vi "Write_output_file.vi"(0 "Output filename":path, 1 "Header":string, 2 "Template Filename":path, 5 "Channel Names":string[](array[string]), 7 "Data":string[][](array[string]), 9 "Desired Columns":i32[](array[numeric])=[0, 1, 2, 3, 4, 5, 6, 7, 8, 9, 10, 11, 12, 13, 14, 15, 16, 17, 18, 19, 20, 21, 22, 23, 24, 25, 26, 27, 28, 29, 30, 31, 32, 33, 34, 35, 36, 37, 38, 39, 40, 41, 42, 43, 44, 45, 46, 47, 48, 49, 50, 51, 52, 53, 54, 55, 56, 57, 58, 59, 60, 61, 62, 63, 64, 65, 66, 67, 68, 69, 70, 71, 72, 73, 74, 75, 76, 77, 78, 79, 80, 81, 82, 83, 84, 85, 86, 87, 88, 89, 90, 91, 92, 93, 94, 95, 96, 97, 98, 99, 100, 101, 102, 103, 104, 105, 106, 107, 108, 109, 110, 111, 112, 113, 114, 115, 116, 117, 118, 119, 120, 121, 122, 123, 124, 125, 126, 127, 128, 129, 130, 131, 132, 133, 134, 135, 136, 137, 138, 139, 140, 141, 142, 143, 144, 145, 146, 147, 148, 149, 150, 151, 152, 153, 154, 155, 156, 157, 158, 159, 160, 161, 162, 163, 164, 165, 166, 167, 168, 169, 170, 171, 172, 173, 174, 175, 176, 177, 178, 179, 180, 181, 182, 183, 184, 185, 186, 187, 188, 189, 190, 191, 192, 193, 194, 195, 196, 197, 198, 199, 200, 201, 202, 203, 204, 205, 206, 207, 208, 209, 210, 211, 212, 213, 214, 215, 216, 217, 218, 219, 220, 221, 222, 223, 224, 225, 226, 227, 228, 229, 230, 231, 232, 233, 234], 11 "Simple Save?":bool, 12 "Save Plotted rows only?":bool, 13 "Summarise mode":T2(ring), 14 "Grouping info":T3[](array[typedef]), 15 "Channels to Tabulate in header":i32[](listbox)) -> (4 "Output filename Out":path)   [LabVIEW 2015]
uses:
  Controls/Group_Binning.ctl
  Results_plotter_Global.vi
panel:
  out "Which Button?":T1(ring)=enum."Center Button"
  out "Table Values":string[][](array[string])
  out "Table Names":string[](array[string])
  out "Table":string
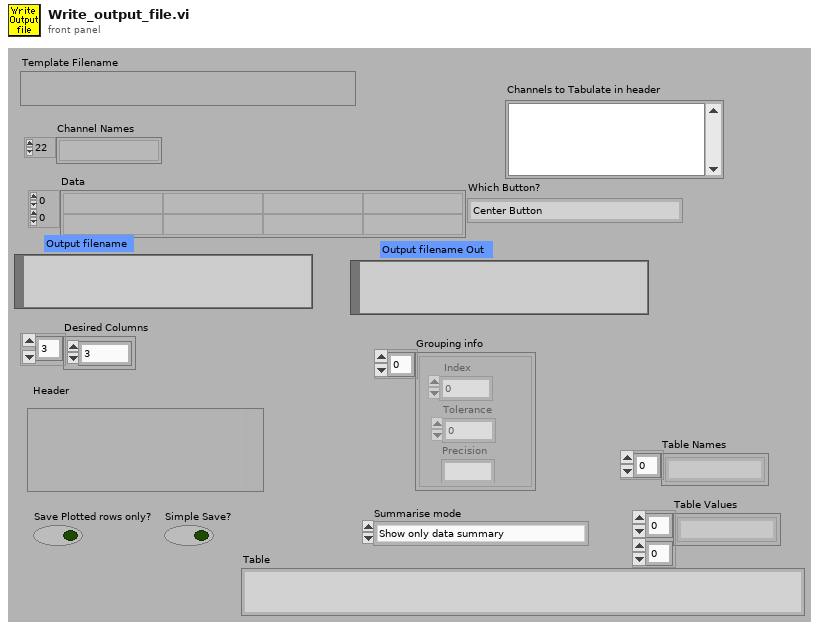
[diagram p1: front panel]
types:
  T1 = enum16{"Left Button", "Center Button", "Right Button", "Window Close"}
  T2 = enum16{"Show only data summary", "Show data summary", "No data summary"}
  T3 = typedef "Group_Binning.ctl" = cluster{"Index":i32, "Tolerance":dbl, "Precision":string}
  T4 = enum32{"existing file", "new file", "new or existing file", "existing dir", "new dir", "new or existing dir", "existing file (use LLBs)", "new file (use LLBs)", "new or existing file (use LLBs)", "new or existing file or directory (use LLBs)"}
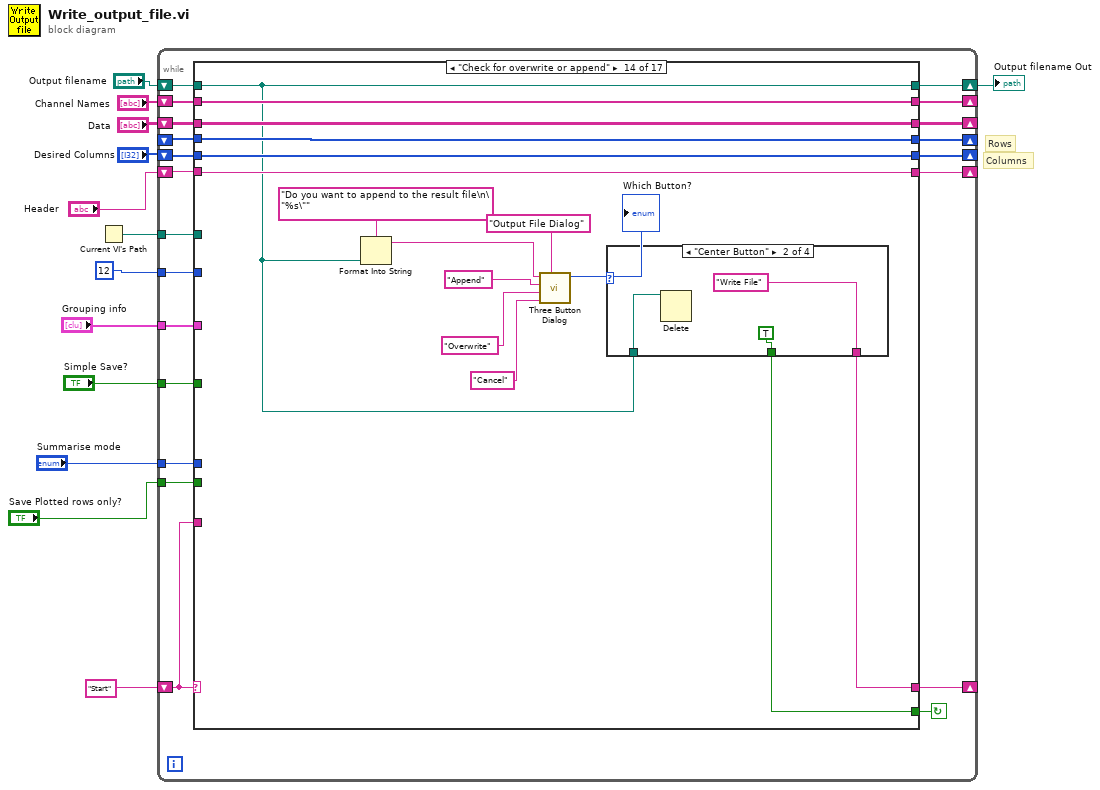
[diagram p0: block diagram]
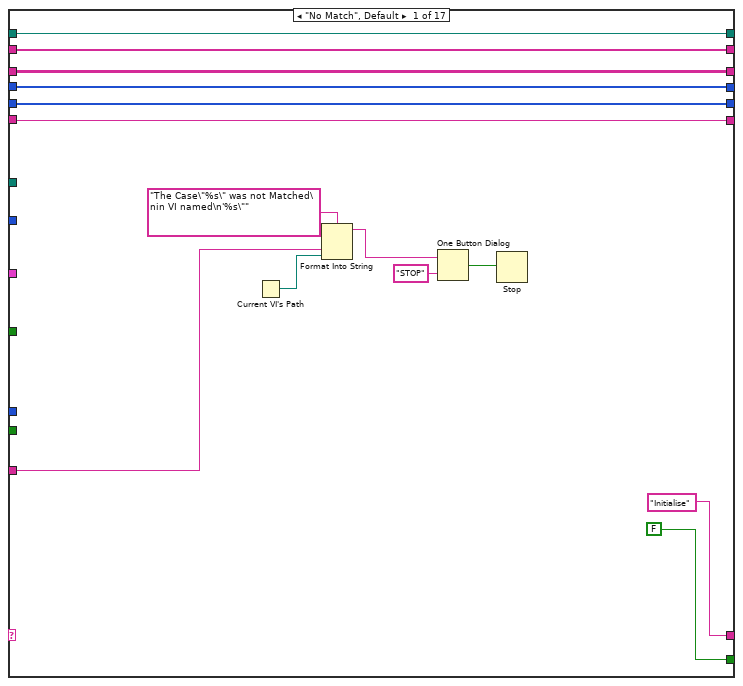
[diagram p2: hidden frame]
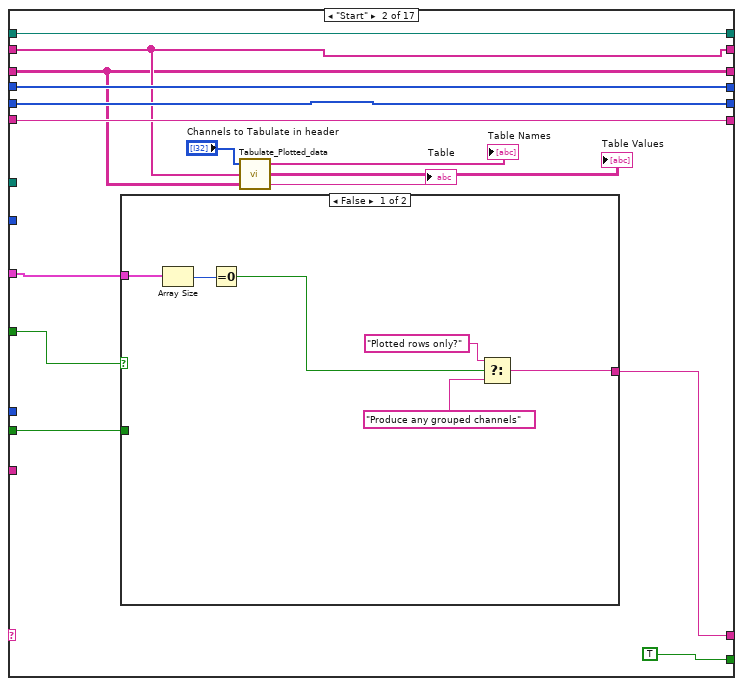
[diagram p3: hidden frame]
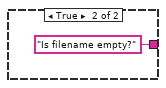
[diagram p4: hidden frame]
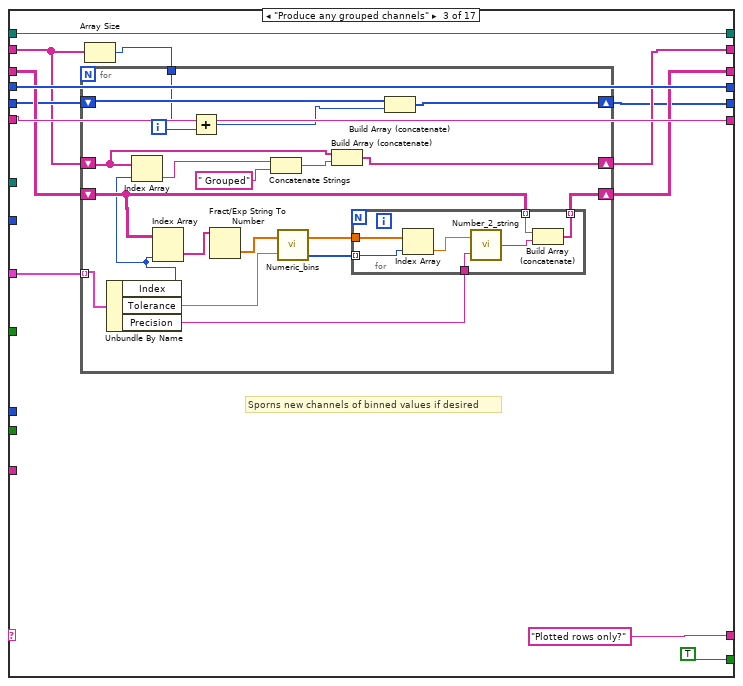
[diagram p5: hidden frame]
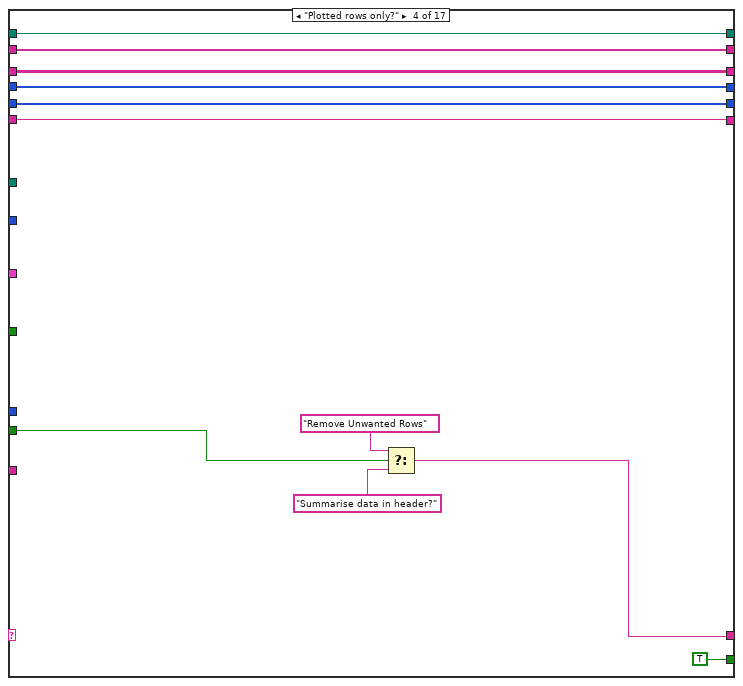
[diagram p6: hidden frame]
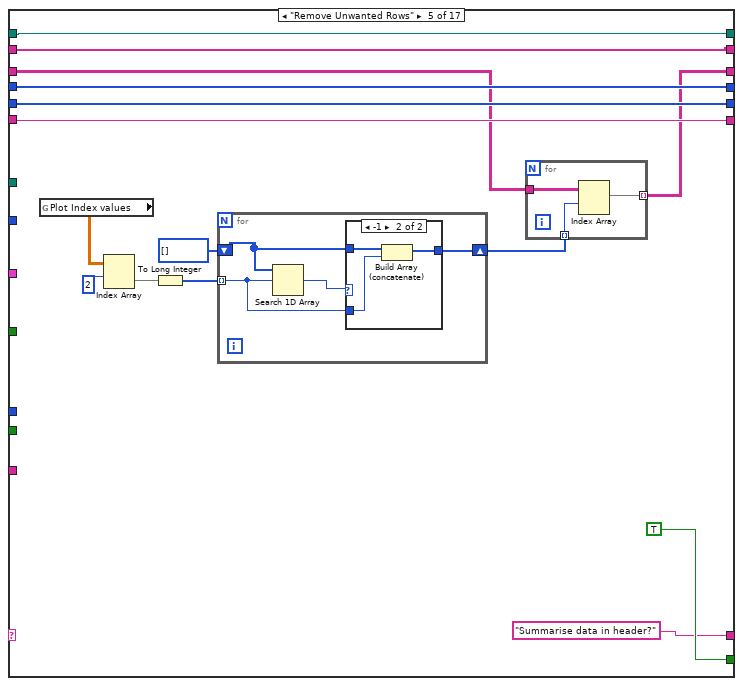
[diagram p7: hidden frame]
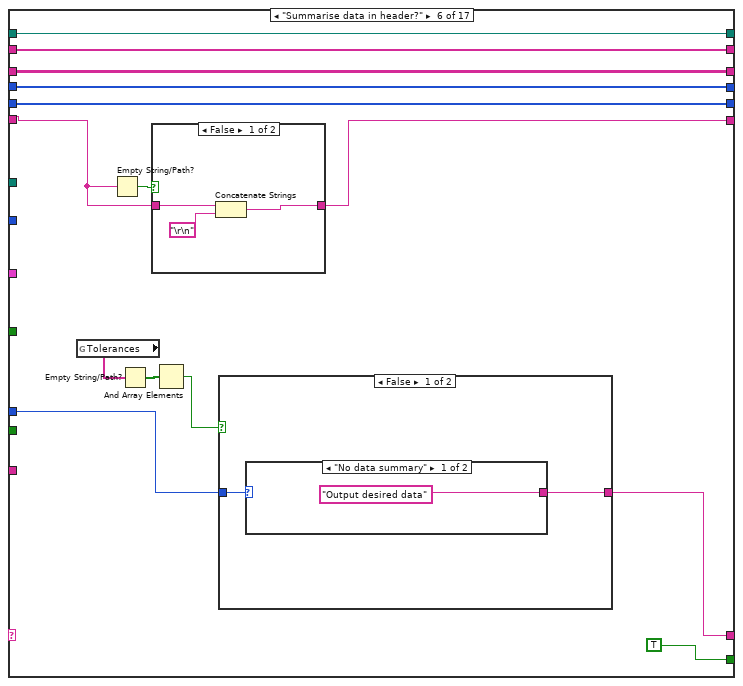
[diagram p9: hidden frame]
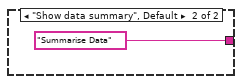
[diagram p10: hidden frame]
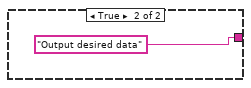
[diagram p11: hidden frame]
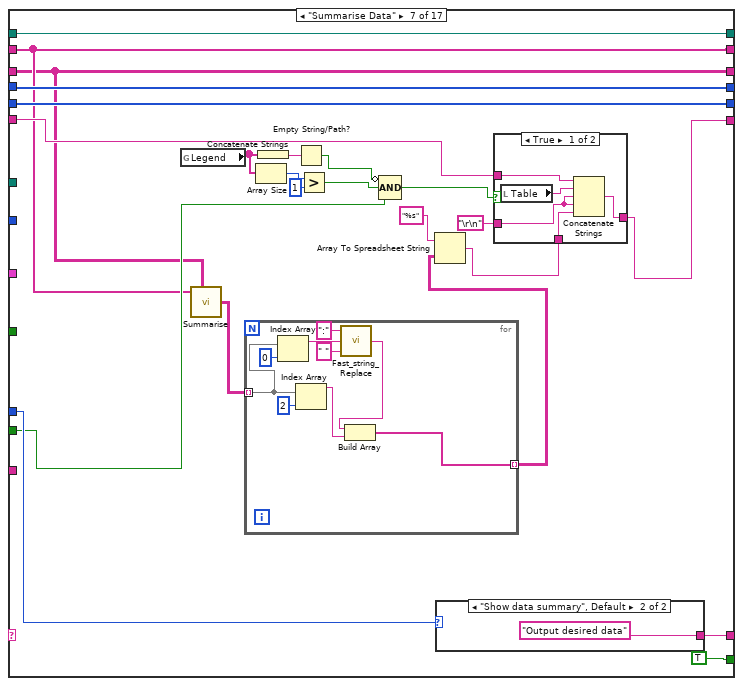
[diagram p13: hidden frame]
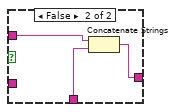
[diagram p14: hidden frame]
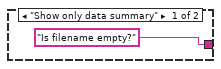
[diagram p15: hidden frame]
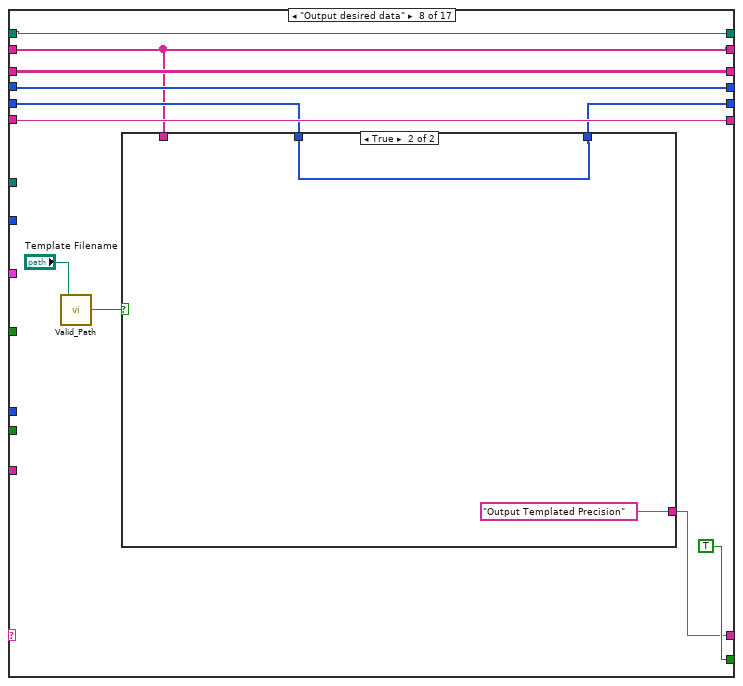
[diagram p16: hidden frame]
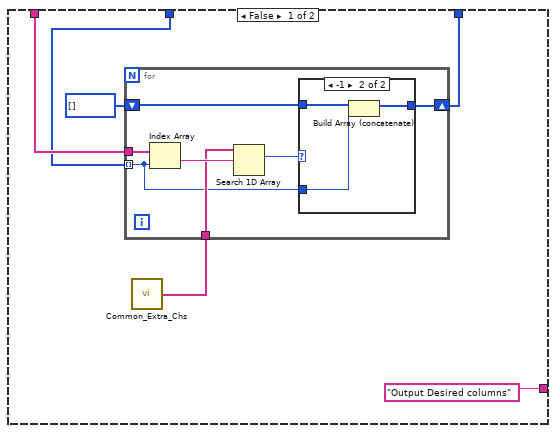
[diagram p17: hidden frame]
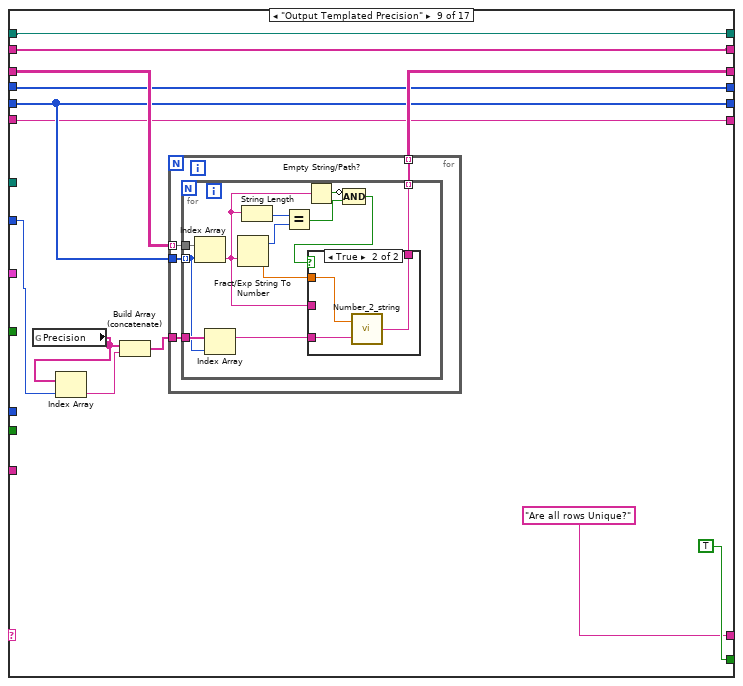
[diagram p19: hidden frame]
diagram:
  # "Columns"
  # "Rows"
  n1 = Current VI's Path() -> (path=w11:path)
  n2 = while {
    shift-left: "Header" -> [w24]
    shift-right: [w27] -> _
    shift-left: "Desired Columns" -> [w26]
    shift-right: [w25] -> _
    shift-left: _ -> [w28]
    shift-right: [w29] -> _
    shift-left: "Data" -> [w31]
    shift-right: [w30] -> _
    shift-left: "Start" -> [w32]
    shift-right: [w33] -> _
    tunnel: w11 -> [w23]
    shift-right: [w22] -> w10
    shift-left: "Output filename" -> [w21]
    shift-right: [w19] -> _
    shift-left: "Channel Names" -> [w20]
    tunnel: "Simple Save?" -> [w18]
    tunnel: 12 ("disabled index (col)") -> [w17]
    tunnel: "Grouping info" -> [w16]
    tunnel: "Summarise mode" -> [w15]
    tunnel: "Save Plotted rows only?" -> [w14]
    stop <- w34 continue-if-true
    n3 = case shown="\"Check for overwrite or append\"" w32 {
      tunnel: [FALSE TRUE TRUE TRUE ("cancelled") TRUE TRUE TRUE TRUE TRUE TRUE TRUE TRUE w349 w366 TRUE ("cancelled") FALSE ("cancelled") FALSE] -> w34
      tunnel: ["Initialise" w60 "Plotted rows only?" w112 "Summarise data in header?" w159 w189 w220 "Are all rows Unique?" "Is filename empty?" w296 "Is filename empty?" w350 w367 "Write File" "End" "End"] -> w33
      tunnel: w32 -> [w43 _ _ _ _ _ _ _ _ _ _ _ _ _ _ _ _]
      tunnel: w31 -> [w40 w53 w79 w116 w128 w155 w172 w217 w254 w283 w303 w339 w354 w376 w396 w410 w436]
      tunnel: [w40 w53 w77 w116 w127 w155 w172 w217 w253 w278 w303 w338 w354 w376 w396 w410 w436] -> w30
      tunnel: [w39 w62 w82 w115 w135 w160 w192 w222 w252 w282 w302 w337 w355 w377 w399 w419 w443] -> w29
      tunnel: w28 -> [w39 w62 w82 w115 w135 w160 w192 w222 w252 w282 _ w337 w355 w377 w399 w419 w443]
      tunnel: [w37 w61 w80 w113 w134 w151 w190 w221 w250 w280 w294 w334 w356 w378 w391 w420 w435] -> w27
      tunnel: w26 -> [w38 w57 w75 w114 w133 w154 w191 w219 w251 w281 w295 w335 w357 w379 w394 w401 w442]
      tunnel: [w38 w57 w72 w114 w133 w154 w191 w218 w251 w281 w295 w335 w357 w379 w394 w401 w442] -> w25
      tunnel: w24 -> [w37 w61 w80 w113 w134 w152 w174 w221 w250 w280 w294 w334 w356 w378 w389 w420 w435]
      tunnel: w23 -> [_ _ _ _ _ _ _ _ _ _ _ _ _ _ _ _ _]
      tunnel: [w36 w59 w81 w118 w123 w158 w188 w216 w248 w277 w293 w333 w353 w365 w393 w406 w438] -> w22
      tunnel: w21 -> [w36 w59 w81 w118 w123 w158 w188 w216 w248 w277 w293 w333 w346 w365 w393 w406 w438]
      tunnel: w20 -> [w35 w54 w74 w117 w122 w156 w173 w215 w247 w276 w292 w332 w348 w374 w395 w403 w439]
      tunnel: [w35 w54 w76 w117 w122 w156 w173 w215 w247 w276 w292 w332 w348 w374 w395 w403 w439] -> w19
      tunnel: w18 -> [_ w58 _ _ _ _ _ _ _ _ _ _ _ _ _ w402 w437]
      tunnel: w17 -> [_ _ _ _ _ _ _ _ w246 _ _ _ _ _ _ _ _]
      tunnel: w16 -> [_ w51 w78 _ _ _ _ _ _ _ _ _ _ _ _ _ _]
      tunnel: w15 -> [_ _ _ _ _ w157 w187 _ _ _ _ _ _ _ _ _ w434]
      tunnel: w14 -> [_ w56 _ w120 _ _ w186 _ _ _ _ _ _ _ _ _ _]
      frame "No Match", Default {
        n4 = Current VI's Path() -> (path=w42:path)
        n5 = Format Into String(format string="The Case\"%s\" was not Matched\nin VI named\n'%s\"" ("Format String"), w43, w42) -> (resulting string=w46:string)  [unwired: 2 in, 1 out]
        n6 = One Button Dialog(message=w46, button name ("OK")="STOP") -> (true=w44:bool)
        n7 = Stop(stop? (T)=w44) -> ()
      }
      frame "Start" {
        n8 = case shown="False" w58 {
          tunnel: [w64 "Is filename empty?" ("f")] -> w60
          tunnel: w56 -> [_ _]
          tunnel: w51 -> [w68 _]
          frame False {
            n9 = Array Size(array=w68) -> (size(s)=w69:i32)
            n10 = Equal To 0?(x=w69) -> (x = 0?=w67:bool)
            n11 = Select(t="Plotted rows only?", s=w67, f="Produce any grouped channels") -> (s? t:f=w64:string)
          }
          frame True {
          }
        }
        n12 = call "Tabulate_Plotted_data.vi"("Data"=w53, "Channel Names"=w54, "Channels to Tabulate"="Channels to Tabulate in header") -> ("spreadsheet string"=→"Table":string, "Channel Values"=→"Table Values":string[][], "Channel Names"=→"Table Names":string[])
      }
      frame "Produce any grouped channels" {
        # "Sporns new channels of binned values if desired"
        n13 = Array Size(array=w74) -> (size(s)=w73:i32)
        n14 = for {
          shift-right: [w95] -> w77
          shift-left: w79 -> [w96]
          tunnel: w78 -> [w100] mode=indexing
          shift-right: [w89] -> w76
          shift-left: w74 -> [w90]
          shift-right: [w87] -> w72
          shift-left: w75 -> [w88]
          tunnel: w73 -> [w85]
          i -> [w86]
          n15 = Unbundle By Name(w100) -> ("Index"=w94:i32, "Tolerance"=w98:dbl, "Precision"=w97:string)
          n16 = Index Array(array=w90, index=w94) -> (element=w92:string)
          n17 = Index Array(array=w96, index (col)=w94) -> (element=w99:string[])  [unwired: 1 in]
          n18 = Add(x=w85, y=w86) -> (x+y=w84:i32)
          n19 = Fract/Exp String To Number(string=w99) -> (number=w103:dbl[])  [unwired: 4 out]
          n20 = Concatenate Strings(w92, " Grouped" ("string")) -> (w91:string)
          n21 = call "Numeric_bins.vi"("Values"=w103, "Tolerance"=w98) -> ("Bin Centres"=w102:dbl[], "Bin Index"=w101:i32[])  [unwired: 1 out]
          n22 = Build Array (concatenate)(w90, w91) -> (w89:string[])
          n23 = for {
            tunnel: w102 -> [w110]
            tunnel: w101 -> [w109] mode=indexing
            tunnel: [w106] -> w95 mode=indexing
            tunnel: w97 -> [w105]
            tunnel: w96 -> [w104] mode=indexing
            n24 = Index Array(array=w110, index=w109) -> (element=w108:dbl)
            n25 = call "Number_2_string.vi"("precision"=w105, "number"=w108) -> ("String"=w107:string)
            n26 = Build Array (concatenate)(w104, w107) -> (w106:string[])
          }
          n27 = Build Array (concatenate)(w88, w84) -> (w87:i32[])
        }
      }
      frame "Plotted rows only?" {
        n28 = Select(t="Remove Unwanted Rows" ("f"), s=w120, f="Summarise data in header?") -> (s? t:f=w112:string)
      }
      frame "Remove Unwanted Rows" {
        n29 = global read "Results_plotter_Global.vi" "Plot Index values"() -> (w132:dbl[][])
        n30 = Index Array(array=w132, index (row)=2 ("disabled index (col)")) -> (element=w131:dbl[])  [unwired: 1 in]
        n31 = To Long Integer(number=w131) -> (32bit integer=w130:i32[])
        n32 = for {
          shift-right: [w141] -> w126
          shift-left: i32[] [] -> [w142]
          tunnel: w130 -> [w140] mode=indexing
          n33 = Search 1D Array(1D array=w142, element=w140) -> (index of element=w143:i32)  [unwired: 1 out]
          n34 = case shown="-1" w143 {
            tunnel: w142 -> [w144 w147]
            tunnel: [w144 w146] -> w141
            tunnel: w140 -> [_ w145]
            frame 0, Default {
            }
            frame -1 {
              n35 = Build Array (concatenate)(w147, w145) -> (w146:i32[])
            }
          }
        }
        n36 = for {
          tunnel: w126 -> [w139] mode=indexing
          tunnel: w128 -> [w138]
          tunnel: [w137] -> w127 mode=indexing
          n37 = Index Array(array=w138, index (row)=w139) -> (element=w137:string[])  [unwired: 1 in]
        }
      }
      frame "Summarise data in header?" {
        n38 = global read "Results_plotter_Global.vi" "Tolerances"() -> (w150:string[])
        n39 = Empty String/Path?(string/path=w152) -> (empty?=w153:bool)
        n40 = Empty String/Path?(string/path=w150) -> (empty?=w149:bool[])
        n41 = case shown="False" w153 {
          tunnel: [w167 w170] -> w151
          tunnel: w152 -> [w168 w170]
          frame False {
            n42 = Concatenate Strings(w168, "\r\n") -> (w167:string)
          }
          frame True {
          }
        }
        n43 = And Array Elements(Boolean array=w149) -> (logical AND=w148:bool)
        n44 = case shown="False" w148 {
          tunnel: [w163 "Output desired data" ("t")] -> w159
          tunnel: w157 -> [w162 _]
          frame False {
            n45 = case shown="\"No data summary\"" w162 {
              tunnel: ["Output desired data" ("t") "Summarise Data"] -> w163
              frame "No data summary" {
              }
              frame "Show data summary", Default {
              }
            }
          }
          frame True {
          }
        }
      }
      frame "Summarise Data" {
        n46 = global read "Results_plotter_Global.vi" "Legend"() -> (w179:string[])
        n47 = call "Summarise.vi"("Channel Names"=w173, "Data"=w172) -> ("Summary"=w184:string[][])  [unwired: 2 in, 1 out]
        n48 = for {
          tunnel: w184 -> [w208] mode=indexing
          tunnel: [w202] -> w171 mode=indexing
          n49 = Index Array(array=w208, index=0) -> (element=w206:string)
          n50 = Index Array(array=w208, index=2) -> (element=w207:string)
          n51 = call "Fast_string_Replace.vi"("Replace match with:"=" ", "Input String"=w206, "regular expression"=":") -> ("Output String"=w203:string)  [unwired: 2 out]
          n52 = Build Array(w203, w207) -> (w202:string[])
        }
        n53 = Array Size(array=w179) -> (size(s)=w178:i32)
        n54 = Concatenate Strings(w179) -> (w181:string)
        n55 = Empty String/Path?(string/path=w181) -> (empty?=w176:bool)
        n56 = Greater?(x=w178, y=1) -> (0:w175:bool)
        n57 = Compound Arithmetic op=AND(invert w176, w175, w186) -> (w180:bool)
        n58 = Array To Spreadsheet String(array=w171, 3:"%s" ("format string")) -> (spreadsheet string=w183:string)  [unwired: 1 out]
        n59 = case shown="\"Show data summary\", Default" w187 {
          tunnel: ["Is filename empty?" "Output desired data"] -> w189
          frame "Show only data summary" {
          }
          frame "Show data summary", Default {
          }
        }
        n60 = case shown="True" w180 {
          tunnel: [w195 w200] -> w190
          tunnel: w174 -> [w198 w199]
          tunnel: w183 -> [w196 w201]
          tunnel: "\r\n" -> [w197 _]
          frame True {
            n61 = local read "Table"() -> (w194:string)
            n62 = Concatenate Strings(w198, w194, w197, w197, w196) -> (w195:string)
          }
          frame False {
            n63 = Concatenate Strings(w199, w201) -> (w200:string)
          }
        }
      }
      frame "Output desired data" {
        n64 = call "Valid_Path.vi"("Filename"="Template Filename") -> ("Valid Path?"=w213:bool)
        n65 = case shown="True" w213 {
          tunnel: ["Output Desired columns" "Output Templated Precision" ("f")] -> w220
          tunnel: w219 -> [w227 w241]
          tunnel: [w225 w241] -> w218
          tunnel: w215 -> [w228 _]
          frame False {
            n66 = call "Common_Extra_Chs.vi"() -> ("Common Extra Channels"=w224:string[])
            n67 = for {
              shift-right: [w230] -> w225
              shift-left: i32[] [] -> [w232]
              tunnel: w228 -> [w236]
              tunnel: w227 -> [w231] mode=indexing
              tunnel: w224 -> [w234]
              n68 = Index Array(array=w236, index=w231) -> (element=w235:string)
              n69 = Search 1D Array(1D array=w234, element=w235) -> (index of element=w233:i32)  [unwired: 1 out]
              n70 = case shown="-1" w233 {
                tunnel: w232 -> [w237 w240]
                tunnel: w231 -> [_ w239]
                tunnel: [w237 w238] -> w230
                frame 0, Default {
                }
                frame -1 {
                  n71 = Build Array (concatenate)(w240, w239) -> (w238:i32[])
                }
              }
            }
          }
          frame True {
          }
        }
      }
      frame "Output Templated Precision" {
        n72 = global read "Results_plotter_Global.vi" "Precision"() -> (w245:string[])
        n73 = Index Array(array=w245, index=w246) -> (element=w243:string)
        n74 = Build Array (concatenate)(w245, w243) -> (w244:string[])
        n75 = for {
          tunnel: w251 -> [w259]
          tunnel: w254 -> [w258] mode=indexing
          tunnel: w244 -> [w257]
          tunnel: [w256] -> w253 mode=indexing
          n76 = for {
            tunnel: w259 -> [w269] mode=indexing
            tunnel: w258 -> [w271]
            tunnel: w257 -> [w270]
            tunnel: [w263] -> w256 mode=indexing
            n77 = Index Array(array=w271, index=w269) -> (element=w262:string)
            n78 = Index Array(array=w270, index=w269) -> (element=w261:string)
            n79 = Fract/Exp String To Number(string=w262) -> (offset past number=w267:i32, number=w264:dbl)  [unwired: 3 out]
            n80 = String Length(string=w262) -> (length=w268:i32)
            n81 = Equal?(x=w268, y=w267) -> (x = y?=w265:bool)
            n82 = Empty String/Path?(string/path=w262) -> (empty?=w266:bool)
            n83 = Compound Arithmetic op=AND(invert w266, w265) -> (w260:bool)
            n84 = case shown="True" w260 {
              tunnel: w261 -> [_ w274]
              tunnel: w264 -> [_ w275]
              tunnel: [w272 w273] -> w263
              tunnel: w262 -> [w272 _]
              frame False {
              }
              frame True {
                n85 = call "Number_2_string.vi"("precision"=w274, "number"=w275) -> ("String"=w273:string)
              }
            }
          }
        }
      }
      frame "Output Desired columns" {
        n86 = for {
          tunnel: w281 -> [w287]
          tunnel: w283 -> [w286] mode=indexing
          tunnel: [w285] -> w278 mode=indexing
          n87 = for {
            tunnel: w287 -> [w289] mode=indexing
            tunnel: w286 -> [w290]
            tunnel: [w288] -> w285 mode=indexing
            n88 = Index Array(array=w290, index=w289) -> (element=w288:string)
          }
        }
      }
      frame "Are all rows Unique?" {
        n89 = for {
          shift-right: [w309] -> _
          shift-left: _ -> [w308]
          tunnel: w303 -> [w311] mode=indexing
          shift-right: [w307] -> w302
          shift-left: _ -> [w306]
          tunnel: [w305] -> w299
          i -> [w305]
          n90 = Array To Spreadsheet String(array=w311, 3:"%s" ("format string")) -> (spreadsheet string=w310:string)  [unwired: 1 out]
          n91 = case shown="0" w305 {
            tunnel: w310 -> [w316 w322]
            tunnel: [w315 w319] -> w309
            tunnel: w308 -> [_ w323]
            tunnel: [w313 w320] -> w307
            tunnel: w306 -> [_ w321]
            tunnel: w305 -> [_ w317]
            frame 0 {
              n92 = Build Array(w316) -> (w315:string[])
              n93 = Build Array(0) -> (w313:i32[])
            }
            frame 1, Default {
              n94 = Search 1D Array(1D array=w323, element=w322) -> (index of element=w318:i32)  [unwired: 1 out]
              n95 = case shown="-1" w318 {
                tunnel: w323 -> [w325 w331]
                tunnel: w322 -> [_ w330]
                tunnel: w321 -> [w324 w329]
                tunnel: [w324 w328] -> w320
                tunnel: [w325 w327] -> w319
                tunnel: w317 -> [_ w326]
                frame 0, Default {
                }
                frame -1 {
                  n96 = Build Array (concatenate)(w331, w330) -> (w327:string[])
                  n97 = Build Array (concatenate)(w329, w326) -> (w328:i32[])
                }
              }
            }
          }
        }
        n98 = Array Size(array=w302) -> (size(s)=w301:i32)
        n99 = Decrement(x=w301) -> (x-1=w300:i32)
        n100 = Equal?(x=w300, y=w299) -> (x = y?=w291:bool)
        n101 = Select(t="Is filename empty?", s=w291, f="Remove Duplicate Rows") -> (s? t:f=w296:string)
      }
      frame "Remove Duplicate Rows" {
        n102 = for {
          tunnel: w337 -> [w343] mode=indexing
          tunnel: w339 -> [w342]
          tunnel: [w341] -> w338 mode=indexing
          n103 = Index Array(array=w342, index (row)=w343) -> (element=w341:string[])  [unwired: 1 in]
        }
      }
      frame "Is filename empty?" {
        n104 = call "Append_Suffiix.vi"("Results file"=w346) -> ("appended path"=w345:path)
        n105 = call "Valid_Path.vi"("Filename"=w345) -> ("Valid Path?"=w347:bool)
        n106 = case shown="False" w347 {
          tunnel: [w358 w364] -> w353
          tunnel: w345 -> [_ w364]
          tunnel: [w360 TRUE ("cancelled")] -> w349
          frame False {
            (unwired) T4."new or existing file" ("select mode (2)")
            n107 = File Dialog(7:"Save Output file as:" ("prompt")) -> (1:w361:bool, 3:w359:path)  [unwired: 1 in, 7 out]
            n108 = Not(x=w361) -> (.not. x?=w360:bool)
            n109 = call "Append_Suffiix.vi"("Results file"=w359) -> ("appended path"=w358:path)
          }
          frame True {
          }
        }
        n110 = call "Does_file_exist_(simple).vi"("Pathname"=w353) -> ("exists?"=w352:bool)
        n111 = Select(t="Check for overwrite or append", s=w352, f="Write File") -> (s? t:f=w350:string)
      }
      frame "Check for overwrite or append" {
        n112 = Format Into String(format string="Do you want to append to the result file\n\"%s\"" ("message"), w365) -> (resulting string=w372:string)  [unwired: 2 in, 1 out]
        n113 = call <vilib>:"Three Button Dialog.vi"("Window Title (\"\")"="Output File Dialog" ("Window Title (\"\")"), "Right Button Text (\"Cancel\")"="Cancel" ("Button 3 Name"), "Center Button Text (\"No\")"="Overwrite" ("F button name (\"Cancel\")"), "Left Button Text (\"Yes\")"="Append" ("T button name (\"OK\")"), "message"=w372) -> ("Which Button?"=w373:T1)  [unwired: 6 out]
        "Which Button?" <- w373
        n114 = case shown="\"Center Button\"" w373 {
          tunnel: ["Append to Results file" ("t") "Write File" "End" ("t") "End"] -> w367
          tunnel: [TRUE TRUE FALSE FALSE] -> w366
          tunnel: w365 -> [_ w382 _ _]
          frame "Left Button" {
          }
          frame "Center Button" {
            n115 = Delete(path (use dialog)=w382) -> ()  [unwired: 4 in, 3 out]
          }
          frame "Right Button" {
          }
          frame "Window Close" {
          }
        }
      }
      frame "Append to Results file" {
        w390 = "\r\n"
        n116 = call "Read_File_Simple.vi"("Filename"=w393) -> ("string"=w392:string)  [unwired: 2 in, 7 out]
        n117 = Concatenate Strings(w392, w390, w390, w390, w389) -> (w391:string)
      }
      frame "Append and Merge Results file" {
        w407 = TRUE  # Read Channel Names only
        w409 = FALSE  # Append last row only
        w413 = TRUE  # exists?
        w416 = FALSE  # Present Channels only
        n118 = case shown="False" w402 {
          tunnel: w401 -> [w423 _]
          tunnel: w403 -> [w422 w427]
          tunnel: [w421 w427] -> w400
          frame False {
            n119 = for {
              tunnel: w423 -> [w424] mode=indexing
              tunnel: w422 -> [w426]
              tunnel: [w425] -> w421 mode=indexing
              n120 = Index Array(array=w426, index=w424) -> (element=w425:string)
            }
          }
          frame True {
          }
        }
        n121 = call "Read_Data_file.vi"("Results file"=w406, "Read Channel Names only"=w407, "Template File"=path "") -> ("String Before"=w405:string)  [unwired: 2 in, 14 out]
        n122 = String Length(string=w405) -> (length=w404:i32)
        n123 = call "Check_and_rewrite_file.vi"("Filename"=w406, "Present Channels only"=w416, "Present Channels"=w400, "Start of read offset (chars.: 0)"=w404) -> ("Merged Channels"=w415:string[], "Merged?"=w414:bool)  [unwired: 10 out]
        n124 = case shown="False" w414 {
          tunnel: [w429 w431] -> w412
          tunnel: w400 -> [w429 w433]
          tunnel: w410 -> [w428 w432]
          tunnel: [w428 w430] -> w411
          tunnel: w415 -> [_ w431]
          frame False {
          }
          frame True {
            n125 = call "Merge_2D_values.vi"("Values In"=w432, "Present Channels"=w433, "Desired Channels"=w431) -> ("Values Out"=w430:string[][])
          }
        }
        n126 = call "Write_Ch_data_file.vi"("Append last row only"=w409, "Header string"=w405, "exists?"=w413, "Channel Values"=w411, "Channel names"=w412, "Filename"=w406) -> ()  [unwired: 1 in, 5 out]
      }
      frame "Write File" {
        n127 = case shown="\"Show data summary\", Default" w434 {
          tunnel: w442 -> [_ w465]
          tunnel: w439 -> [_ w464]
          tunnel: w438 -> [w448 w462]
          tunnel: w437 -> [_ w459]
          tunnel: w436 -> [_ w457]
          tunnel: w435 -> [_ w455]
          frame "Show only data summary" {
            w449 = FALSE  # Present Channels only
            n128 = local read "Table Names"() -> (w447:string[])
            n129 = local read "Which Button?"() -> (w445:T1)
            n130 = call "Check_and_rewrite_file.vi"("Filename"=w448, "Present Channels only"=w449, "Present Channels"=w447) -> ("Merged Channels"=w450:string[])  [unwired: 1 in, 11 out]
            n131 = case shown="\"Center Button\"" w445 {
              tunnel: [w451 FALSE ("exists?")] -> w444
              frame "Left Button", Default {
                w451 = TRUE  # exists?
              }
              frame "Center Button" {
              }
            }
            n132 = local read "Table Values"() -> (w446:string[][])
            n133 = call "Write_Ch_data_file.vi"("exists?"=w444, "Channel Values"=w446, "Channel names"=w450, "Filename"=w448) -> ()  [unwired: 4 in, 4 out]
          }
          frame "Show data summary", Default {
            w461 = FALSE  # Append last row only
            w463 = FALSE  # exists?
            n134 = global read "Results_plotter_Global.vi" "Description"() -> (w453:string[])
            n135 = Empty String/Path?(string/path=w455) -> (empty?=w454:bool)
            n136 = case shown="True" w459 {
              tunnel: w465 -> [w472 _]
              tunnel: w453 -> [w471 _]
              tunnel: [w467 w478] -> w456
              tunnel: w464 -> [w470 w479]
              tunnel: [w469 w479] -> w458
              tunnel: w457 -> [w466 w478]
              frame False {
                n137 = for {
                  tunnel: w472 -> [w474] mode=indexing
                  tunnel: w470 -> [w477]
                  tunnel: [w476] -> w469 mode=indexing
                  tunnel: w471 -> [w475]
                  tunnel: [w473] -> w468 mode=indexing
                  n138 = Index Array(array=w477, index=w474) -> (element=w476:string)
                  n139 = Index Array(array=w475, index=w474) -> (element=w473:string)
                }
                n140 = Build Array (concatenate)(w468, w466) -> (w467:string[][])
              }
              frame True {
              }
            }
            n141 = case shown="False" w454 {
              tunnel: [w482 ""] -> w460
              tunnel: w455 -> [w480 _]
              frame False {
                n142 = Initialize Array("", 10 ("Dimension Size")) -> (w485:string[])
                n143 = call "Asterisk_header.vi"("Channel names"=w485) -> ("Header string"=w484:string)
                n144 = Concatenate Strings(w480, "\r\n", "#" ("Substring"), w484) -> (w482:string)
              }
              frame True {
              }
            }
            n145 = call "Write_Ch_data_file.vi"("Append last row only"=w461, "Header string"=w460, "exists?"=w463, "Channel Values"=w456, "Channel names"=w458, "Filename"=w462) -> ()  [unwired: 1 in, 5 out]
          }
        }
      }
    }
  }
  "Output filename Out" <- w10
